vi "Create.vi"(8 "error in":errorcluster, 9 "Z":dbl, 10 "Y":dbl, 11 "X":dbl) -> (0 "error out":errorcluster, 3 "Vec3d Class out":refnum<class "Vec3d Class.lvclass">)   [LabVIEW 2011, in "Vec3d Class.lvclass"]
uses:
  Vec3d Class.lvclass
  Vec3d Class.lvclass/Vec3d Class.ctl
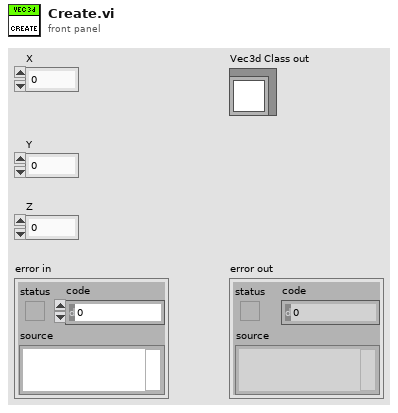
[diagram p1: front panel]
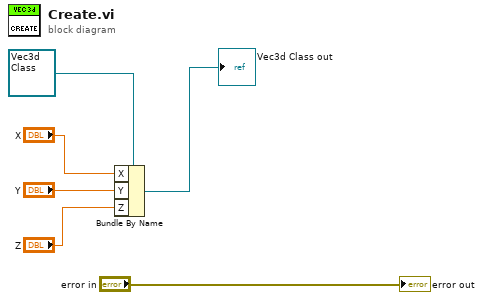
[diagram p0: block diagram]
diagram:
  n1 = Bundle By Name(cluster=refnum<class "Vec3d Class.lvclass"> refnum ("Vec3d Class in"), "X"="X", "Y"="Y", "Z"="Z") -> (→"Vec3d Class out":refnum<class "Vec3d Class.lvclass">)
  "error out" <- "error in"
